vi "Interpolate_ArrayTable_Polynomial.vi"(6 "algorithm":T1 items=["SVD", "Givens", "Givens2", "Householder", "LU Decomposition", "Cholesky", "SVD for Rank Deficient H"], 7 "array":dbl[][](array[numeric]), 9 "method":T2 items=["Least Square", "Least Absolute Residual", "Bisquare"], 11 "Desired_Distance":dbl) -> (1 "Polynomial Coefficients":dbl[](array[numeric]), 2 "Best Polynomial Fit":dbl[](array[numeric]), 3 "RPM":dbl)   [LabVIEW 2019]
uses:
  <vilib>/Analysis/6fits.llb/Curve Fitting Criteria.ctl
  <vilib>/Analysis/6fits.llb/General Linear Fit Algorithm.ctl
  <vilib>/Analysis/polynomials.llb/Scalar Polynomial Evaluation (DBL).vi
  <vilib>/Analysis/NI_AALPro.lvlib
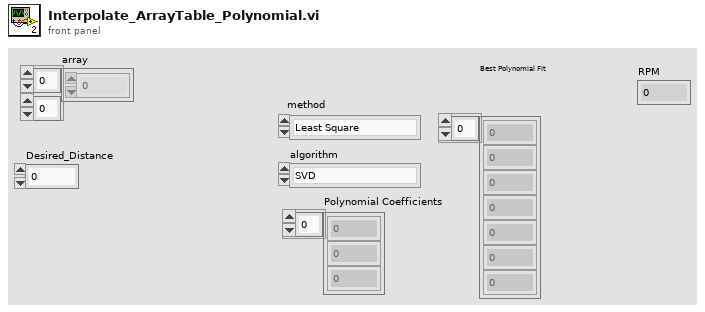
[diagram p1: front panel]
types:
  T1 = typedef "NI_AALPro.lvlib/General Linear Fit Algorithm.ctl" = u16
  T2 = typedef "NI_AALPro.lvlib/Curve Fitting Criteria.ctl" = u16
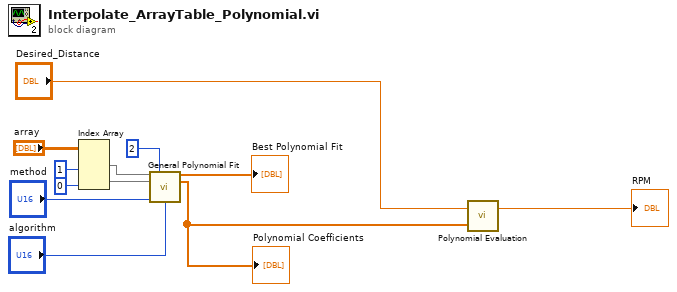
[diagram p0: block diagram]
diagram:
  n1 = Index Array(array="array", index (col) #1=1 ("disabled index (col)"), index (col) #2=0 ("index (col)")) -> (element #1=w4:dbl[], element #2=w5:dbl[])  [unwired: 2 in]
  n2 = call <vilib>:"General Polynomial Fit.vi"("Y"=w4, "polynomial order"=2, "X"=w5, "method"="method", "algorithm"="algorithm") -> ("Best Polynomial Fit"=→"Best Polynomial Fit":dbl[], "Polynomial Coefficients"=w2:dbl[])  [unwired: 7 in, 2 out]
  "Polynomial Coefficients" <- w2
  n3 = call-poly <vilib>:"Polynomial Evaluation.vi"("P(x)"=w2, "a"="Desired_Distance") -> ("P(a)"=→"RPM":dbl)  [unwired: 1 out]
